vi "Station Calibration.vi"() -> ()   [LabVIEW 2017]
uses:
  Shared Components/Gantry Class/Type Definitions/Virtual Modes.ctl
  Shared Components/Utils/Type Definitions/Object Types.ctl
  Shared Components/Gantry Class/Type Definitions/Init_Modes.ctl
  Shared Components/Gantry Class/Gantry Class.lvclass
  Shared Components/Vec3d Class/Vec3d Class.lvclass
panel:
  in  "Results Folder":path=path "C:/Users/Admin/Gantry Purdue/pixel-gantry-control/Results"
  in  "Enum":T1
  in  "Virtual Mode":T2=enum."Virtual"
  in  "stop":bool
  out "Image":T3(plugin-control)
  out "error out":errorcluster
  in  "Config Folder":path=path "C:/Users/Admin/Gantry Purdue/pixel-gantry-control/Config"
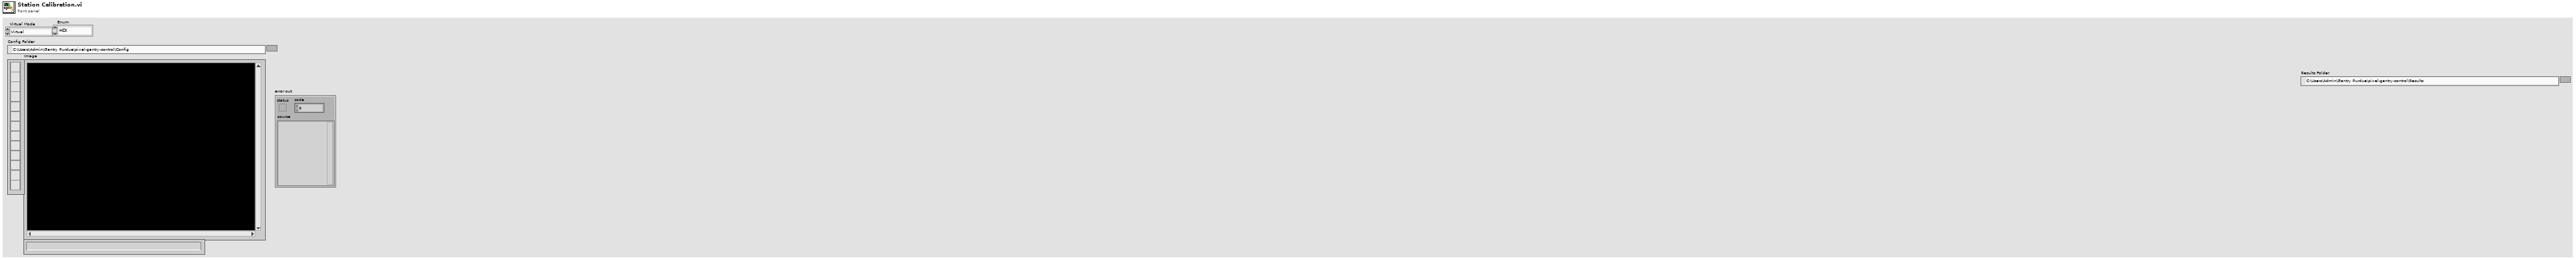
[diagram p1: front panel]
types:
  T1 = typedef "Object Types.ctl" = enum16{"HDI", "Glass Piece", "Other"}
  T2 = typedef "Virtual Modes.ctl" = enum16{"Nonvirtual", "Pseudovirtual", "Virtual"}
  T3 = typedef "IMAQ Image.ctl" = refnum<image>
  T4 = typedef "Init_Modes.ctl" = enum16{"Full", "Robot Only", "Dispenser Only", "Cameras Only", "Robot and Cameras", "Robot and Cameras and Dispenser", "Manifold Only"}
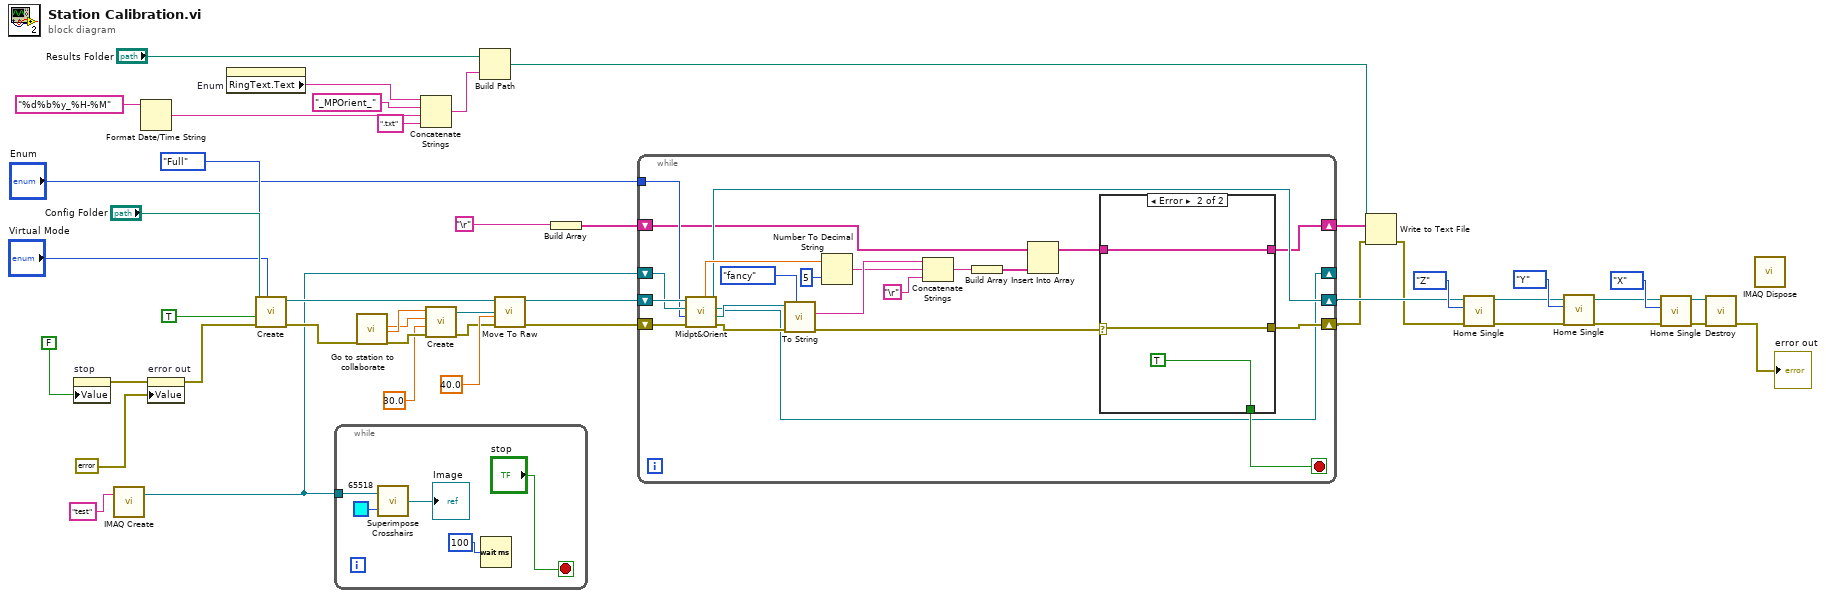
[diagram p0: block diagram]
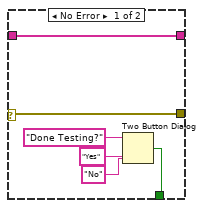
[diagram p2: hidden frame]
diagram:
  n1 = property on="stop" class="Bool (strict)"("Value"=FALSE) -> (error out=w42:errorcluster)  [unwired: 2 in, 1 out]
  n2 = call "IMAQ Create"("Image Name"="test") -> ("New Image"=w25:T3)  [unwired: 4 in, 1 out]
  n3 = Format Date/Time String(time format string (%c)="%d%b%y_%H-%M") -> (date/time string=w10:string)  [unwired: 2 in]
  n4 = property on="error out" class="Clust (strict)"(error in=w42, "Value"=errorcluster {"status"=FALSE, "code"=0, "source"=""} ("error in (no error)")) -> (error out=w41:errorcluster)  [unwired: 1 in, 1 out]
  n5 = property on="Enum" class="Enum (strict)"() -> ("RingText.Text"=w9:string)  [unwired: 2 in, 2 out]
  n6 = call "Create.vi"("Virtual Mode"="Virtual Mode", "error in"=w41, "HOME?"=TRUE, "Config Folder"="Config Folder", "Init Mode"=Init_Modes."Full") -> ("error out"=w38:errorcluster, "Gantry out"=w29:refnum<class "Gantry Class.lvclass">)  [unwired: 5 in]
  n7 = while {
    tunnel: w25 -> [w49]
    stop <- "stop" stop-if-true
    n8 = call "Superimpose Crosshairs.vi"("Grid Line Color"=u32 65518, "Refnum in"=w49) -> ("Refnum out"=→"Image":T3)
    n9 = Wait (ms)(milliseconds to wait=u32 100) -> ()  [unwired: 1 out]
  }
  n10 = call "Go to station to collaborate"("error in (no error)"=w38) -> ("Y"=w36:dbl, "X"=w37:dbl, "error out"=w34:errorcluster)  [unwired: 15 in, 1 out]
  n11 = Concatenate Strings(w9, "_MPOrient_" ("string"), w10, ".txt" ("string")) -> (w12:string)
  n12 = call "Create.vi"("error in"=w34, "Z"=30.0, "Y"=w36, "X"=w37) -> ("error out"=w28:errorcluster, "Vec3d Class out"=w31:refnum<class "Vec3d Class.lvclass">)  [unwired: 6 in]
  n13 = Build Path(base path="Results Folder", name or relative path=w12) -> (appended path=w15:path)
  n14 = call-dynamic "Move To Raw.vi"("error in"=w28, "Speed"=40.0, "Destination"=w31, "Gantry in"=w29) -> ("error out"=w27:errorcluster, "Gantry out"=w26:refnum<class "Gantry Class.lvclass">)  [unwired: 6 in]
  n15 = Build Array("\r" ("string")) -> (w6:string[])
  n16 = while {
    shift-right: [w56] -> _
    shift-left: w25 -> [w71]
    shift-right: [w57] -> w3
    shift-left: w26 -> [w72]
    shift-right: [w62] -> w2
    shift-left: w27 -> [w73]
    tunnel: "Enum" -> [w58]
    shift-right: [w54] -> w4
    shift-left: w6 -> [w55]
    stop <- w61 stop-if-true
    n17 = call-dynamic "Midpt&Orient.vi"("error in (no error)"=w73, "Enum"=w58, "Image In"=w71, "Gantry Class in"=w72) -> ("error out"=w64:errorcluster, "Midpoint"=w70:refnum<class "Vec3d Class.lvclass">, "Image Out"=w56:T3, "Gantry Class out"=w57:refnum<class "Gantry Class.lvclass">, "Orientation"=w67:dbl)  [unwired: 3 in]
    n18 = call "To String.vi"("Formatting"=enum16{"plain", "fancy"}."fancy", "error in"=w64, "Vec3d in"=w70) -> ("error out"=w63:errorcluster, "Vec3d String"=w68:string)  [unwired: 6 in, 1 out]
    n19 = Number To Decimal String(number=w67, width (-)=i16 5) -> (decimal integer string=w66:string)
    n20 = Concatenate Strings(w68, w66, "\r" ("string")) -> (w65:string)
    n21 = Build Array(w65) -> (w60:string[])
    n22 = Insert Into Array(array=w55, new element=w60) -> (w59:string[])  [unwired: 1 in]
    n23 = case shown="Error" w63 {
      selector: w63 -> [w75 w82]
      tunnel: [w75 w82] -> w62
      tunnel: [w76 TRUE ("Done Testing?")] -> w61
      tunnel: w59 -> [w74 w80]
      tunnel: [w74 w80] -> w54
      frame No Error {
        n24 = Two Button Dialog(message="Done Testing?", 1:"No" ("F button name (\"Cancel\")"), 2:"Yes" ("T button name (\"OK\")")) -> (T button?=w76:bool)
      }
      frame Error {
      }
    }
  }
  n25 = Write to Text File(file (use dialog)=w15, text=w4, error in=w2) -> (error out=w1:errorcluster)  [unwired: 1 in, 2 out]
  n26 = call-dynamic "Home Single.vi"("error in"=w1, "Axis"=enum16{"X", "Y", "Z", "U"}."Z", "Gantry in"=w3) -> ("error out"=w20:errorcluster, "Gantry out"=w21:refnum<class "Gantry Class.lvclass">)  [unwired: 7 in]
  n27 = call-dynamic "Home Single.vi"("error in"=w20, "Axis"=enum16{"X", "Y", "Z", "U"}."Y", "Gantry in"=w21) -> ("error out"=w18:errorcluster, "Gantry out"=w19:refnum<class "Gantry Class.lvclass">)  [unwired: 7 in]
  n28 = call-dynamic "Home Single.vi"("error in"=w18, "Axis"=enum16{"X", "Y", "Z", "U"}."X", "Gantry in"=w19) -> ("error out"=w16:errorcluster, "Gantry out"=w17:refnum<class "Gantry Class.lvclass">)  [unwired: 7 in]
  n29 = call "Destroy.vi"("error in"=w16, "Gantry Class in"=w17) -> ("error out"=→"error out":errorcluster)  [unwired: 9 in]
  n30 = call "IMAQ Dispose"() -> ()  [unwired: 6 in, 1 out]
